vi "Create output file.vi"(8 "error in (no error)":errorcluster, 10 "temp file path":path, 11 "PrintToSingleFileHtml in":refnum<class "PrintToSingleFileHtml.lvclass">) -> (0 "error out":errorcluster, 3 "PrintToSingleFileHtml out":refnum<class "PrintToSingleFileHtml.lvclass">)   [LabVIEW 2026, in "PrintToSingleFileHtml.lvclass"]
uses:
  PrintToSingleFileHtml.lvclass
  <vilib>/regexp/Match Regular Expression.xnode
  PrintToSingleFileHtml.lvclass/PrintToSingleFileHtml.ctl
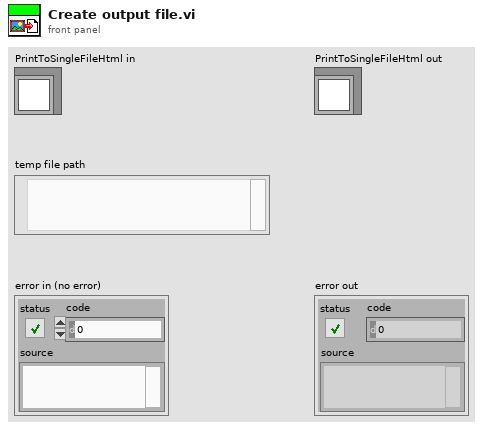
[diagram p1: front panel]
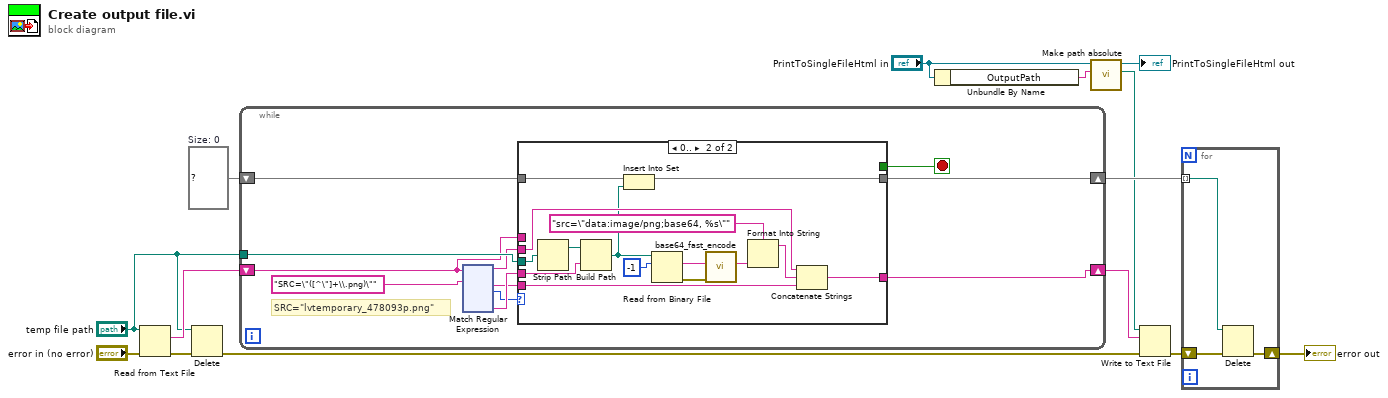
[diagram p0: block diagram]
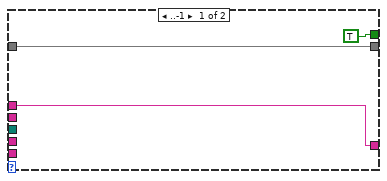
[diagram p2: hidden frame]
diagram:
  w12 = set{path} {}  # Size: 0
  n1 = Read from Text File(file (use dialog)="temp file path", error in="error in (no error)") -> (text=w9:string, error out=w11:errorcluster)  [unwired: 2 in, 2 out]
  n2 = Delete(path (use dialog)="temp file path", error in=w11) -> (error out=w2:errorcluster)  [unwired: 3 in, 2 out]
  n3 = while {
    tunnel: "temp file path" -> [w23]
    shift-right: [w20] -> w10
    shift-left: w9 -> [w18]
    shift-right: [w16] -> w13
    shift-left: w12 -> [w15]
    stop <- w17 stop-if-true
    # "SRC=\"lvtemporary_478093p.png\""
    n4 = xnode "Match Regular Expression"("input string"=w18, "regular expression"="SRC=\"([^\"]+\\.png)\"") -> ("before match"=w22:string, "after match"=w21:string, "offset past match"=w19:i32, "submatch 1"=w24:string)  [unwired: 4 in, 2 out]
    n5 = case shown="0.." w19 {
      tunnel: w24 -> [_ w41]
      tunnel: w23 -> [_ w39]
      tunnel: w22 -> [_ w36]
      tunnel: w21 -> [_ w35]
      tunnel: [w28 w33] -> w20
      tunnel: w18 -> [w28 _]
      tunnel: [TRUE _] -> w17
      tunnel: [w26 w30] -> w16
      tunnel: w15 -> [w26 w29]
      frame ..-1 {
      }
      frame 0.. {
        n6 = Strip Path(path=w39) -> (stripped path=w40:path)  [unwired: 1 out]
        n7 = Build Path(base path=w40, name or relative path=w41) -> (appended path=w31:path)
        n8 = Insert Into Set(10:w31, 11:w29) -> (3:w30:set{path})  [unwired: 1 out]
        n9 = Read from Binary File(10:-1 ("count (1)"), 11:w31) -> (0:w32:errorcluster, 2:w42:string)  [unwired: 4 in, 2 out]
        n10 = call "base64_fast_encode.vi"("error in (no error)"=w32, "string in (not encoded)"=w42) -> ("string out (base64-encoded)"=w37:string)  [unwired: 8 in, 1 out]
        n11 = Format Into String(format string="src=\"data:image/png;base64, %s\"", w37) -> (resulting string=w34:string)  [unwired: 2 in, 1 out]
        n12 = Concatenate Strings(w36, w34, w35) -> (w33:string)
      }
    }
  }
  n13 = Unbundle By Name("PrintToSingleFileHtml in") -> ("OutputPath"=w5:string)
  n14 = call "Make path absolute.vi"("relative or absolute path"=w5, "PrintToSingleFileHtml in"="PrintToSingleFileHtml in") -> ("absolute path"=w3:path, "PrintToSingleFileHtml out"=→"PrintToSingleFileHtml out":refnum<class "PrintToSingleFileHtml.lvclass">)  [unwired: 8 in]
  n15 = Write to Text File(file (use dialog)=w3, text=w10, error in=w2) -> (error out=w14:errorcluster)  [unwired: 1 in, 2 out]
  n16 = for {
    tunnel: w13 -> [w165] mode=indexing
    shift-right: [w163] -> w6
    shift-left: w14 -> [w164]
    n17 = Delete(path (use dialog)=w165, error in=w164) -> (error out=w163:errorcluster)  [unwired: 3 in, 2 out]
  }
  "error out" <- w6
